vi "Sequence.GetSequenceChannels.vi"(6 "Refs":refnum<vi>[](array[refnum]), 8 "error in (no error)":errorcluster, 9 "Aliases Array":string[](array[string]), 10 "Aliases.All":T1[](array[typedef]), 11 "ChannelsLookup":variant) -> (0 "error out":errorcluster, 1 "Warnings":string, 2 "SequenceChannels":T2, 3 "ChannelsLookup":variant)   [LabVIEW 2013, in "Simple Sequence Tools - Editor.lvlib"]
uses:
  Simple Sequence Tools - Editor.lvlib
  Types/Compiled.SequenceChannels.ctl
  Shared/Types/Channel.Properties.ctl
  Shared/Simple Sequence Tools - Shared.lvlib
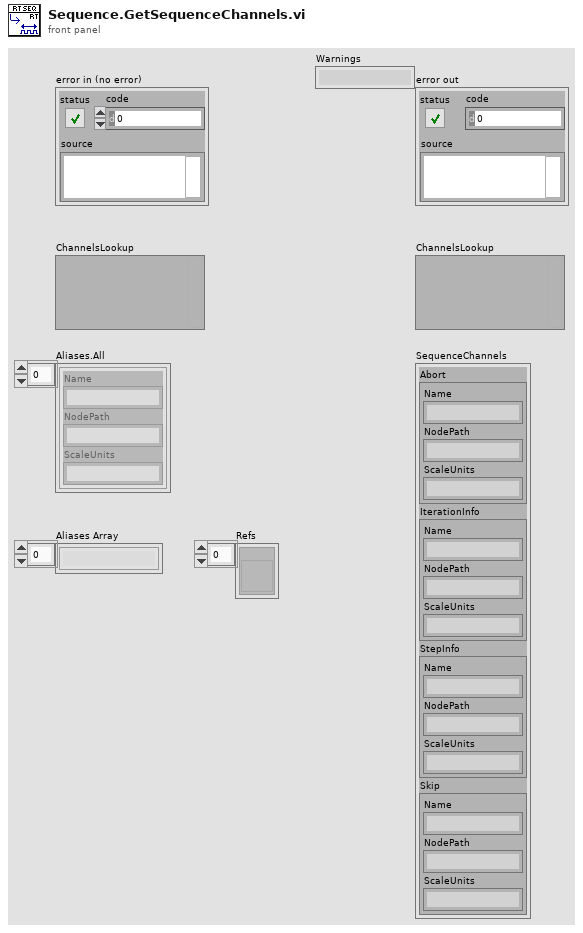
[diagram p1: front panel]
types:
  T1 = typedef "Simple Sequence Tools - Shared.lvlib/Channel.Properties.ctl" = cluster{"Name":string, "NodePath":string, "ScaleUnits":string}
  T2 = typedef "Simple Sequence Tools - Editor.lvlib/Compiled.SequenceChannels.ctl" = cluster{"Abort":T1, "IterationInfo":T1, "StepInfo":T1, "Skip":T1}
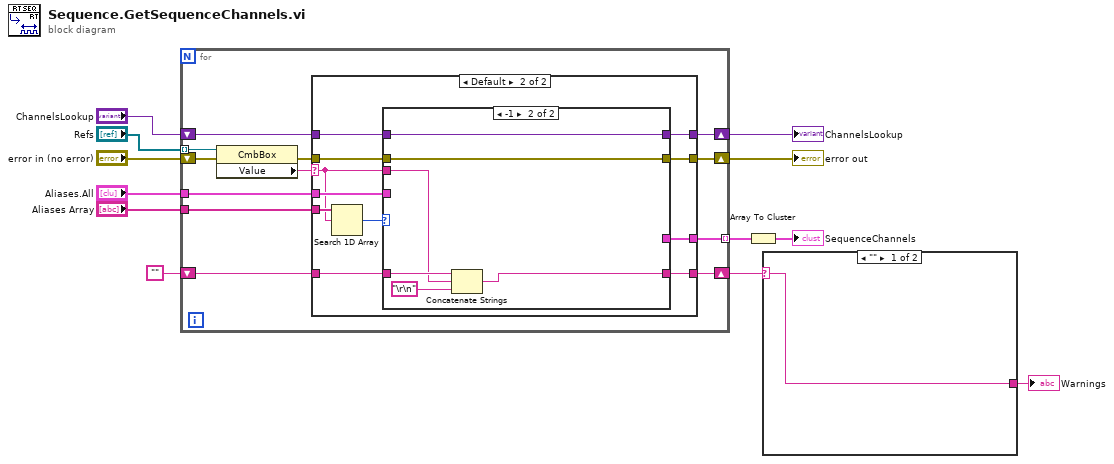
[diagram p0: block diagram]
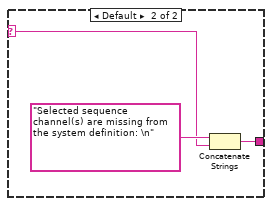
[diagram p2: hidden frame]
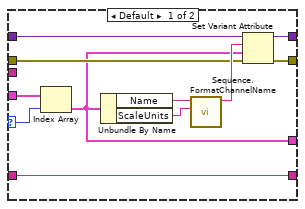
[diagram p4: hidden frame]
diagram:
  n1 = for {
    tunnel: "Refs" -> [w23] mode=indexing
    shift-right: [w19] -> w4
    shift-left: "error in (no error)" -> [w24]
    tunnel: "Aliases.All" -> [w21]
    tunnel: "Aliases Array" -> [w22]
    shift-right: [w17] -> w12
    shift-left: "ChannelsLookup" -> [w18]
    tunnel: [w16] -> w8 mode=indexing
    shift-right: [w14] -> w1
    shift-left: "" -> [w13]
    n2 = property class="CmbBox"(reference=w23, error in=w24) -> (error out=w20:errorcluster, "Value"=w15:string)  [unwired: 1 out]
    n3 = case shown="Default" w15 {
      selector: w15 -> [_ w30]
      tunnel: w22 -> [_ w38]
      tunnel: w21 -> [_ w36]
      tunnel: w20 -> [w27 w35]
      tunnel: [w27 w34] -> w19
      tunnel: w18 -> [w26 w33]
      tunnel: [w26 w32] -> w17
      tunnel: [_ w31] -> w16
      tunnel: [w25 w29] -> w14
      tunnel: w13 -> [w25 w28]
      frame "" {
      }
      frame Default {
        n4 = Search 1D Array(1D array=w38, element=w30) -> (index of element=w37:i32)  [unwired: 1 in]
        n5 = case shown="-1" w37 {
          selector: w37 -> [w48 _]
          tunnel: w36 -> [w49 _]
          tunnel: w35 -> [w44 w54]
          tunnel: [w43 w54] -> w34
          tunnel: w33 -> [w42 w55]
          tunnel: [w41 w55] -> w32
          tunnel: [w40 _] -> w31
          tunnel: w30 -> [_ w51]
          tunnel: [w39 w53] -> w29
          tunnel: w28 -> [w39 w52]
          frame Default {
            n6 = Index Array(array=w49, index=w48) -> (element=w40:T1)
            n7 = Unbundle By Name(w40) -> ("Name"=w46:string, "ScaleUnits"=w45:string)
            n8 = call "Sequence.FormatChannelName.vi"("ScaleUnits"=w45, "Name"=w46) -> ("ChannelName"=w47:string)  [unwired: 9 in]
            n9 = Set Variant Attribute(Variant=w42, name=w47, value=w40, error in=w44) -> (Variant out=w41:variant, error out=w43:errorcluster)  [unwired: 1 out]
          }
          frame -1 {
            n10 = Concatenate Strings(w52, w51, "\r\n") -> (w53:string)
          }
        }
      }
    }
  }
  "ChannelsLookup" <- w12
  "error out" <- w4
  n11 = Array To Cluster(array=w8) -> (cluster=→"SequenceChannels":cluster{"[0]":T1, "[1]":T1, "[2]":T1, "[3]":T1})
  n12 = case shown="\"\"" w1 {
    selector: w1 -> [w56 w57]
    tunnel: [w56 w58] -> w2
    frame "" {
    }
    frame Default {
      n13 = Concatenate Strings("Selected sequence channel(s) are missing from the system definition: \n" ("format string"), w57) -> (w58:string)
    }
  }
  "Warnings" <- w2
